vi "decodeExtType.vi"(8 "error in (no error)":errorcluster, 9 "BinaryArray":u8[](array[numeric]) format="%x", 10 "Variant In":variant) -> (0 "error out":errorcluster, 2 "Variant Out":variant, 5 "Type":string)   [LabVIEW 2015, in "MsgPack.lvlib"]
uses:
  MsgPack.lvlib
  <vilib>/ErrorRing/Error Ring.xnode
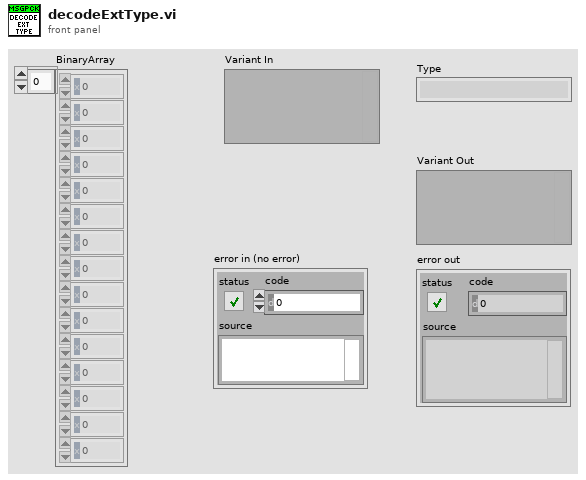
[diagram p1: front panel]
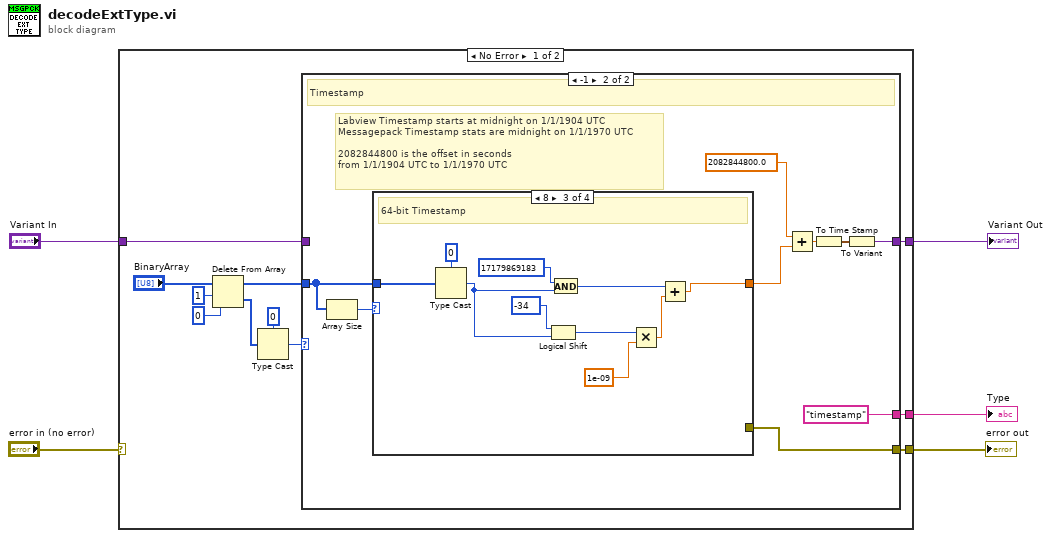
[diagram p0: block diagram]
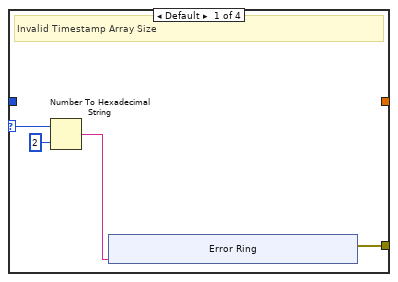
[diagram p3: hidden frame]
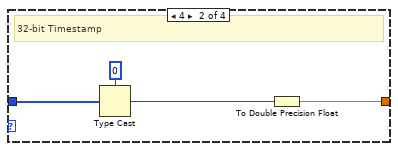
[diagram p4: hidden frame]
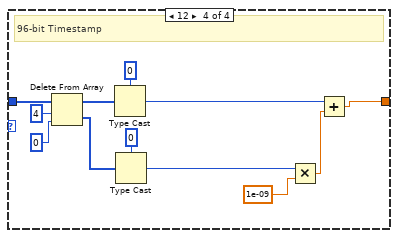
[diagram p5: hidden frame]
diagram:
  n1 = case shown="No Error" "error in (no error)" {
    selector: "error in (no error)" -> [_ w63]
    tunnel: [w13 w63] -> w5
    tunnel: [w16 _] -> w1
    tunnel: [w14 w62] -> w2
    tunnel: "Variant In" -> [w15 w62]
    frame No Error {
      n2 = Delete From Array(array="BinaryArray", length=1, index=0) -> (deleted portion=w8:u8[], array with subset deleted=w11:u8[])
      n3 = Type Cast(type=i8 0, x=w8) -> (*(type *) &x=w7:i8)
      n4 = case shown="-1" w7 {
        tunnel: [_ "timestamp"] -> w16
        tunnel: w15 -> [w17 _]
        tunnel: [w17 w21] -> w14
        tunnel: w11 -> [_ w22]
        tunnel: [_ w24] -> w13
        frame Default {
          # "Undefined Ext Type"
        }
        frame -1 {
          # "Labview Timestamp starts at midnight on 1/1/1904 UTC\nMessagepack Timestamp stats are midnight on 1/1/1970 UTC\n\n2082844800 is the offset in seconds\nfrom 1/1/1904 UTC to 1/1/1970 UTC"
          # "Timestamp"
          n5 = Array Size(array=w22) -> (size(s)=w25:i32)
          n6 = case shown="8" w25 {
            selector: w25 -> [w29 _ _ _]
            tunnel: [w28 _ _ _] -> w24
            tunnel: w22 -> [_ w39 w49 w57]
            tunnel: [_ w36 w43 w60] -> w19
            frame Default {
              # "Invalid Timestamp Array Size"
              n7 = Number To Hexadecimal String(1:i16 2 ("width (-)"), 2:w29) -> (0:w27:string)
              n8 = xnode "Error Ring"("parameter 0"=w27) -> ("error out"=w28:errorcluster)
            }
            frame 4 {
              # "32-bit Timestamp"
              n9 = Type Cast(type=u32 0, x=w39) -> (*(type *) &x=w37:u32)
              n10 = To Double Precision Float(number=w37) -> (double precision float=w36:dbl)
            }
            frame 8 {
              # "64-bit Timestamp"
              n11 = Type Cast(type=u64 0, x=w49) -> (*(type *) &x=w46:u64)
              n12 = Logical Shift(y=i16 -34 ("x"), x=w46) -> (x << y=w41:u64)
              n13 = And(x=u64 17179869183, y=w46) -> (x .and. y?=w44:u64)
              n14 = Multiply(x=w41, y=1e-09) -> (x*y=w42:dbl)
              n15 = Add(x=w44, y=w42) -> (x+y=w43:dbl)
            }
            frame 12 {
              # "96-bit Timestamp"
              n16 = Delete From Array(array=w57, length=4, index=0) -> (deleted portion=w51:u8[], array with subset deleted=w54:u8[])
              n17 = Type Cast(type=i64 0, x=w54) -> (*(type *) &x=w53:i64)
              n18 = Type Cast(type=u32 0, x=w51) -> (*(type *) &x=w50:u32)
              n19 = Multiply(x=w50, y=1e-09) -> (x*y=w59:dbl)
              n20 = Add(x=w53, y=w59) -> (x+y=w60:dbl)
            }
          }
          n21 = Add(x=2082844800.0 ("y"), y=w19) -> (x+y=w23:dbl)
          n22 = To Time Stamp(1:w23) -> (0:w20:timestamp)
          n23 = To Variant(anything=w20) -> (Variant=w21:variant)
        }
      }
    }
    frame Error {
    }
  }
  "error out" <- w5
  "Variant Out" <- w2
  "Type" <- w1
